vi "Robot Main.vi"() -> ()   [LabVIEW 2014]
doc: "This VI implements the framework and scheduler for your robotics program. It should not be necessary to modify the framework. You are expected to add your code to the VIs called from Robot Main - the ones located in the Team Code folder within the project."
uses:
  <vilib>/Rock Robotics/WPI/MotorControl/WPI_MotorControlDeviceRef.ctl
  <vilib>/Rock Robotics/WPI/MotorControl/WPI_MotorControlType.ctl
  <vilib>/Rock Robotics/SystemInterfaces/Typedef/FPGA_TypedefDigitalModule.ctl
  <vilib>/Rock Robotics/SystemInterfaces/DIO/FPGA_DIOPWMChannel.ctl
  <vilib>/Rock Robotics/WPI/PWM/WPI_PWMDeadband.ctl
  <vilib>/Rock Robotics/WPI/CAN/Jaguar/SubVIs/WPI_CANJaguar_ControlMode.ctl
  <vilib>/Rock Robotics/WPI/CAN/TalonSRX/WPI_CANTalonSRX_APIControlMode.ctl
  <vilib>/Rock Robotics/WPI/PWM/WPI_PWMTransform_ConPane.ctl
  <vilib>/Rock Robotics/WPI/Switch/WPI_SwitchDevRef.ctl
  <vilib>/Rock Robotics/SystemInterfaces/DIO/FPGA_DIOChannel.ctl
  <vilib>/Rock Robotics/SystemInterfaces/Counter/FPGA_CounterCtrSystemIndex.ctl
  <vilib>/Rock Robotics/SystemInterfaces/AI/FPGA_AIChannel.ctl
  <vilib>/Rock Robotics/WPI/Joystick/WPI_JoystickDeviceEnum.ctl
  <vilib>/Rock Robotics/WPI/MotorControl/WPI_MotorControlOpen Talon.vi
  <vilib>/Rock Robotics/WPI/Switch/WPI_SwitchOpenLimit.vi
  <vilib>/Rock Robotics/WPI/MotorControl/WPI_MotorControlOpen Victor.vi
  <vilib>/Rock Robotics/WPI/Counter/WPI_CounterDigitalInputToDigitalSource.vi
  <vilib>/Rock Robotics/WPI/RobotDrive/WPI_RobotDriveOpen4MotorWithVictor.vi
  Robot Global Data.vi
panel:
  in  "Gains DOWN":cluster{"P":dbl, "I":dbl, "D":dbl}={"P"=0.15555, "I"=5.6e-07, "D"=0.0}
  out "all currents (A)":dbl[](array[numeric])
  in  "Lift Deadband":dbl=0.1
  in  "Manual?":bool
  out "Distance":dbl
  out "Tolerable?":bool
  in  "Limit":dbl=0.666
  in  "Gains":cluster{"P":dbl, "I":dbl, "D":dbl}={"P"=0.15555, "I"=5.6e-07, "D"=0.0}
  in  "Limit Switches":T5={"Lift Top"={"DevStatus"={"status"=FALSE, "code"=0, "source"=""}, "DIO Channel"=enum."Invalid", "Controller"=enum."Controller 1", "CntIndex"=enum."Invalid", "Normally Closed"=FALSE}, "Lift Bottom"={"DevStatus"={"status"=FALSE, "code"=0, "source"=""}, "DIO Channel"=enum."Invalid", "Controller"=enum."Controller 1", "CntIndex"=enum."Invalid", "Normally Closed"=FALSE}, "Gripper 1"={"DevStatus"={"status"=FALSE, "code"=0, "source"=""}, "DIO Channel"=enum."Invalid", "Controller"=enum."Controller 1", "CntIndex"=enum."Invalid", "Normally Closed"=FALSE}, "Gripper 2"={"DevStatus"={"status"=FALSE, "code"=0, "source"=""}, "DIO Channel"=enum."Invalid", "Controller"=enum."Controller 1", "CntIndex"=enum."Invalid", "Normally Closed"=FALSE}}
  in  "Motors":T14
  # "P = 7\nI = 2.5E -5"
  # "devided gains by 45"
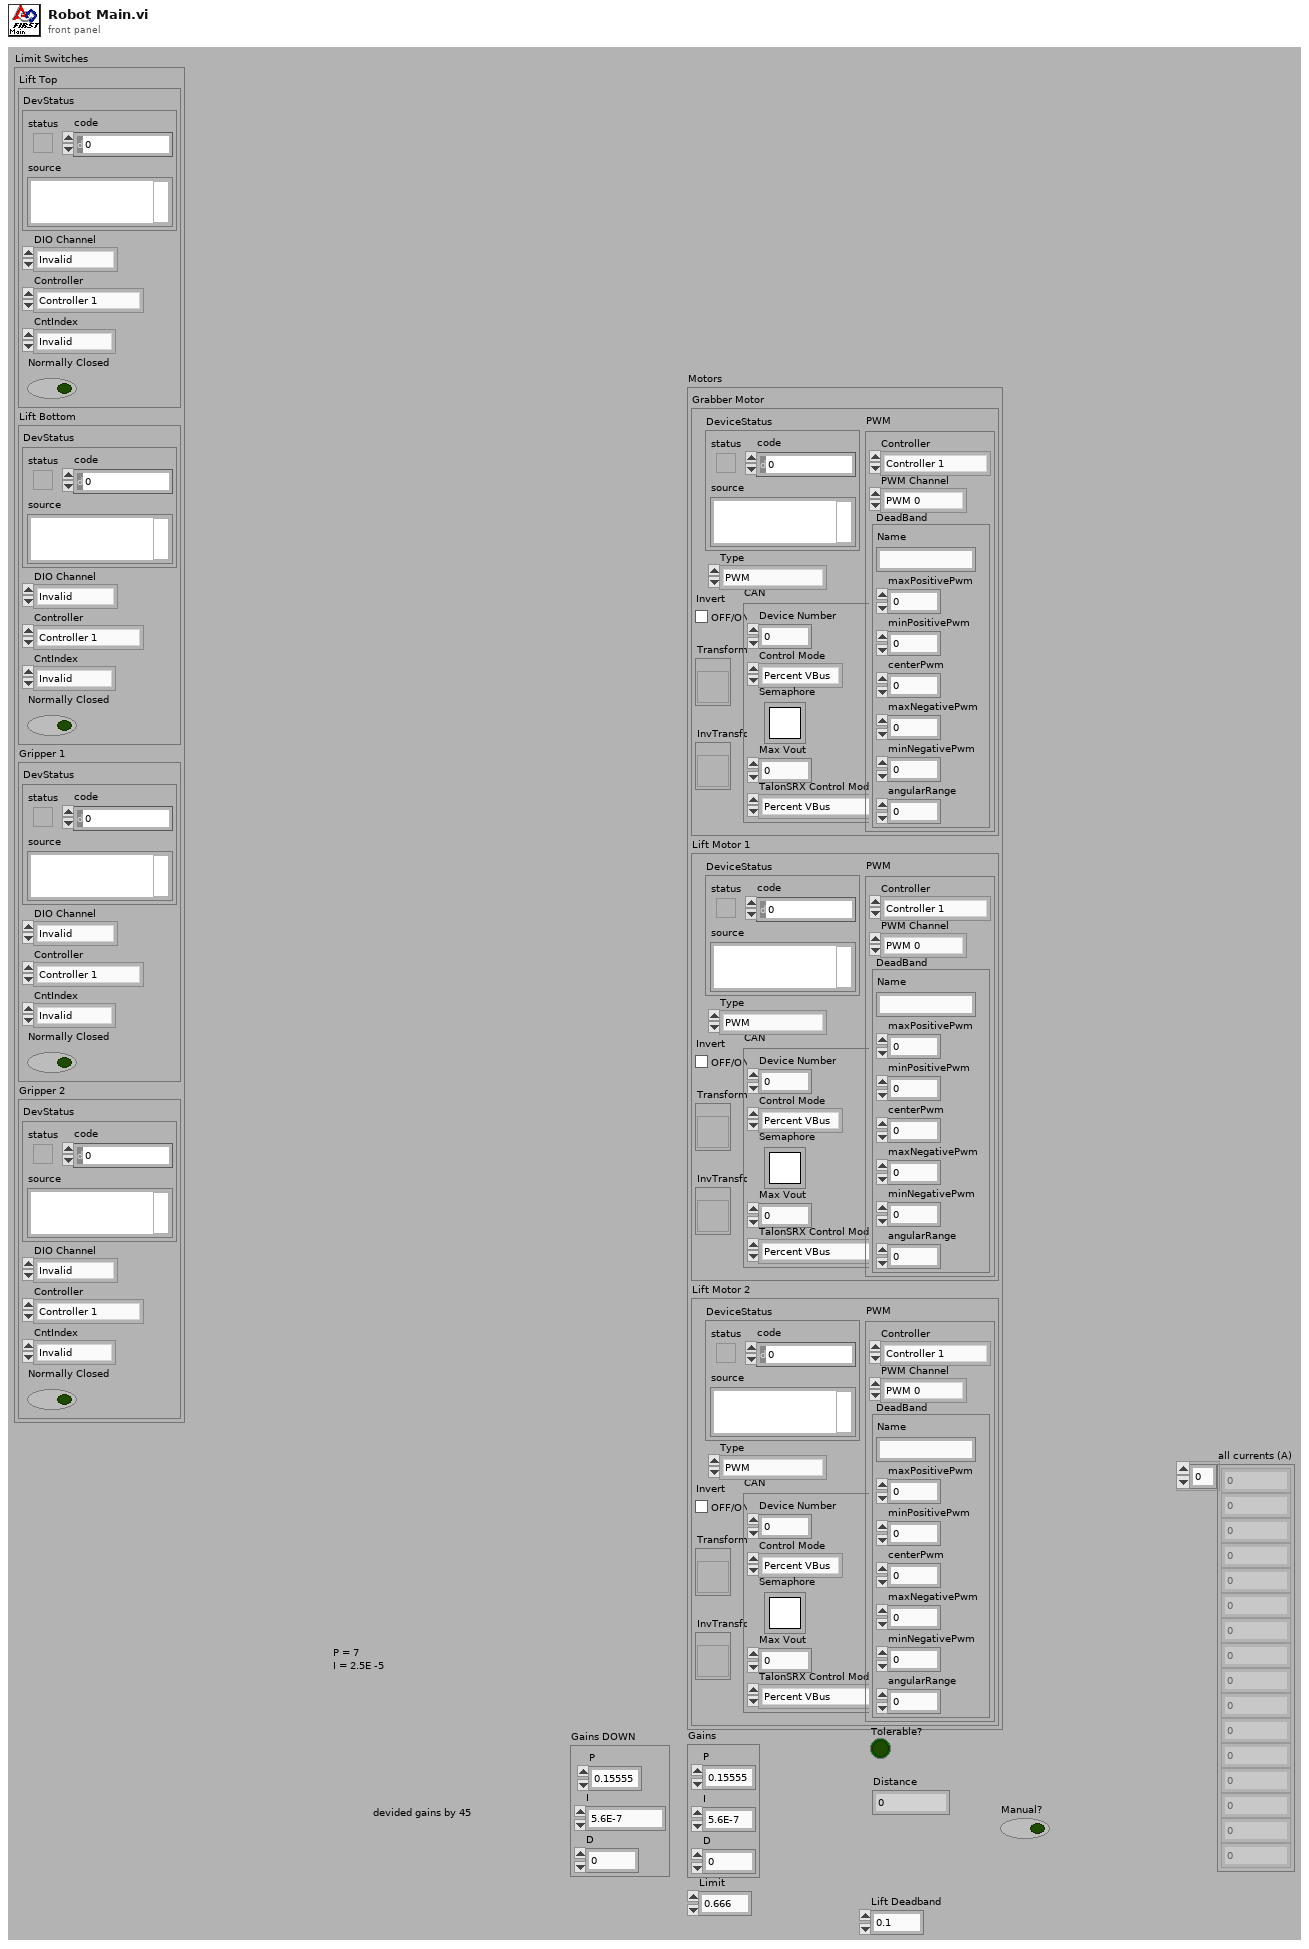
[diagram p1: front panel]
types:
  T1 = typedef "WPI_SwitchDevRef.ctl" = cluster{"DevStatus":errorcluster, "DIO Channel":T2, "Controller":T3, "CntIndex":T4, "Normally Closed":bool}
  T2 = typedef "FPGA_DIOChannel.ctl" = enum8{"DIO 0", "DIO 1", "DIO 2", "DIO 3", "DIO 4", "DIO 5", "DIO 6", "DIO 7", "DIO 8", "DIO 9", "DIO MXP 0", "DIO MXP 1", "DIO MXP 2", "DIO MXP 3", "DIO MXP 4", "DIO MXP 5", "DIO MXP 6", "DIO MXP 7", "DIO MXP 8", "DIO MXP 9", "DIO MXP 10", "DIO MXP 11", "DIO MXP 12", "DIO MXP 13", "DIO MXP 14", "DIO MXP 15", "Invalid"}
  T3 = typedef "FPGA_TypedefDigitalModule.ctl" = enum16{"Controller 1"}
  T4 = typedef "FPGA_CounterCtrSystemIndex.ctl" = enum8{"Ctr 0", "Ctr 1", "Ctr 2", "Ctr 3", "Ctr 4", "Ctr 5", "Ctr 6", "Ctr 7", "Invalid"}
  T5 = cluster{"Lift Top":T1, "Lift Bottom":T1, "Gripper 1":T1, "Gripper 2":T1}
  T6 = typedef "WPI_MotorControlDeviceRef.ctl" = cluster{"DeviceStatus":errorcluster, "Type":T7, "PWM":cluster{"Controller":T3, "PWM Channel":T8, "DeadBand":T9}, "CAN":cluster{"Device Number":u8, "Control Mode":T10, "Semaphore":T11, "Max Vout":dbl, "TalonSRX Control Mode":T12}, "Invert":bool, "TransformRef":T13, "InvTransformRef":T13}
  T7 = typedef "WPI_MotorControlType.ctl" = enum16{"PWM", "CAN", "CANTalonSRX"}
  T8 = typedef "FPGA_DIOPWMChannel.ctl" = enum8{"PWM 0", "PWM 1", "PWM 2", "PWM 3", "PWM 4", "PWM 5", "PWM 6", "PWM 7", "PWM 8", "PWM 9", "PWM MXP 0", "PWM MXP 1", "PWM MXP 2", "PWM MXP 3", "PWM MXP 4", "PWM MXP 5", "PWM MXP 6", "PWM MXP 7", "PWM MXP 8", "PWM MXP 9", "Invalid"}
  T9 = typedef "WPI_PWMDeadband.ctl" = cluster{"Name":string, "maxPositivePwm":i32, "minPositivePwm":i32, "centerPwm":i32, "maxNegativePwm":i32, "minNegativePwm":i32, "angularRange":u16}
  T10 = typedef "WPI_CANJaguar_ControlMode.ctl" = enum8{"Percent VBus", "Current", "Speed", "Position", "Voltage"}
  T11 = typedef "Semaphore RefNum" = refnum<k1>
  T12 = typedef "WPI_CANTalonSRX_APIControlMode.ctl" = enum8{"Percent VBus", "Speed", "Position", "Slave", "Unchanged / Invalid"}
  T13 = typedef "WPI_PWMTransform_ConPane.ctl" = refnum<vi>
  T14 = cluster{"Grabber Motor":T6, "Lift Motor 1":T6, "Lift Motor 2":T6}
  T15 = typedef "WPI_JoystickDeviceEnum.ctl" = enum16{"USB 0", "USB 1", "USB 2", "USB 3", "USB 4", "USB 5"}
  T16 = typedef "FPGA_AIChannel.ctl" = enum8{"AI 0", "AI 1", "AI 2", "AI 3", "AI MXP 0", "AI MXP 1", "AI MXP 2", "AI MXP 3", "Invalid"}
  T17 = typedef "WPI_DigitalInputDevRef.ctl" = cluster{"DevStatus":errorcluster, "DIO Channel":T2, "Controller":T3}
  T18 = typedef "WPI_JoystickDevRef.ctl" = cluster{"Device":T15}
  T19 = typedef "FPGA_CounterEncoderSourceConvertionLVSourceType.ctl" = cluster{"DevStatus":errorcluster, "AnalogTriggerMode?":bool, "DigitalMode":cluster{"Controller":T3, "DIO Channel":T20}, "AnalogTriggerMode":cluster{"AnalogTriggerIndex":T21, "OutputType":T22}}
  T20 = typedef "FPGA_DIODigitalSourceChannel.ctl" = enum8{"DIO 0", "DIO 1", "DIO 2", "DIO 3", "DIO 4", "DIO 5", "DIO 6", "DIO 7", "DIO 8", "DIO 9", "DIO MXP 0", "DIO MXP 1", "DIO MXP 2", "DIO MXP 3", "DIO MXP 4", "DIO MXP 5", "DIO MXP 6", "DIO MXP 7", "DIO MXP 8", "DIO MXP 9", "DIO MXP 10", "DIO MXP 11", "DIO MXP 12", "DIO MXP 13", "DIO MXP 14", "DIO MXP 15", "Disabled"}
  T21 = typedef "FPGA_AnalogTriggerIndex.ctl" = enum8{"Trig 0", "Trig 1", "Trig 2", "Trig 3", "Trig 4", "Trig 5", "Trig 6", "Trig 7", "Invalid"}
  T22 = typedef "FPGA_AnalogTriggerOutType.ctl" = enum16{"InWindow", "TriggerState", "Rising", "Falling"}
  T23 = typedef "WPI_PotentiometerDevRef.ctl" = cluster{"DevStatus":errorcluster, "Controller":T24, "Analog Channel":T16, "Invert Output":bool}
  T24 = typedef "FPGA_TypedefAnalogModule.ctl" = enum16{"Controller 1"}
  T25 = typedef "WPI_EncoderDevRef.ctl" = cluster{"DevStatus":errorcluster, "EncoderIndex":T26, "CounterIndex":T4, "DistancePerCount":dbl, "Decoding Type":T27}
  T26 = typedef "FPGA_EncoderIdx.ctl" = enum8{"Enc 0", "Enc 1", "Enc 2", "Enc 3", "Enc 4", "Enc 5", "Enc 6", "Enc 7", "Invalid"}
  T27 = typedef "WPI_EncoderType.ctl" = enum16{"1x", "2x", "4x"}
  T28 = typedef "WPI_RobotDriveDevRef.ctl" = cluster{"DevStatus":errorcluster, "Motors[]":T6[], "Square Inputs":bool, "Max Output":dbl}
  T29 = typedef "WPI_DriverStationRobotMode2.ctl" = enum16{"Autonomous Disabled", "Autonomous Enabled", "Teleop Disabled", "Teleop Enabled", "Disconnected", "Finish", "Test Disabled", "Test Enabled", "Emergency Stopped"}
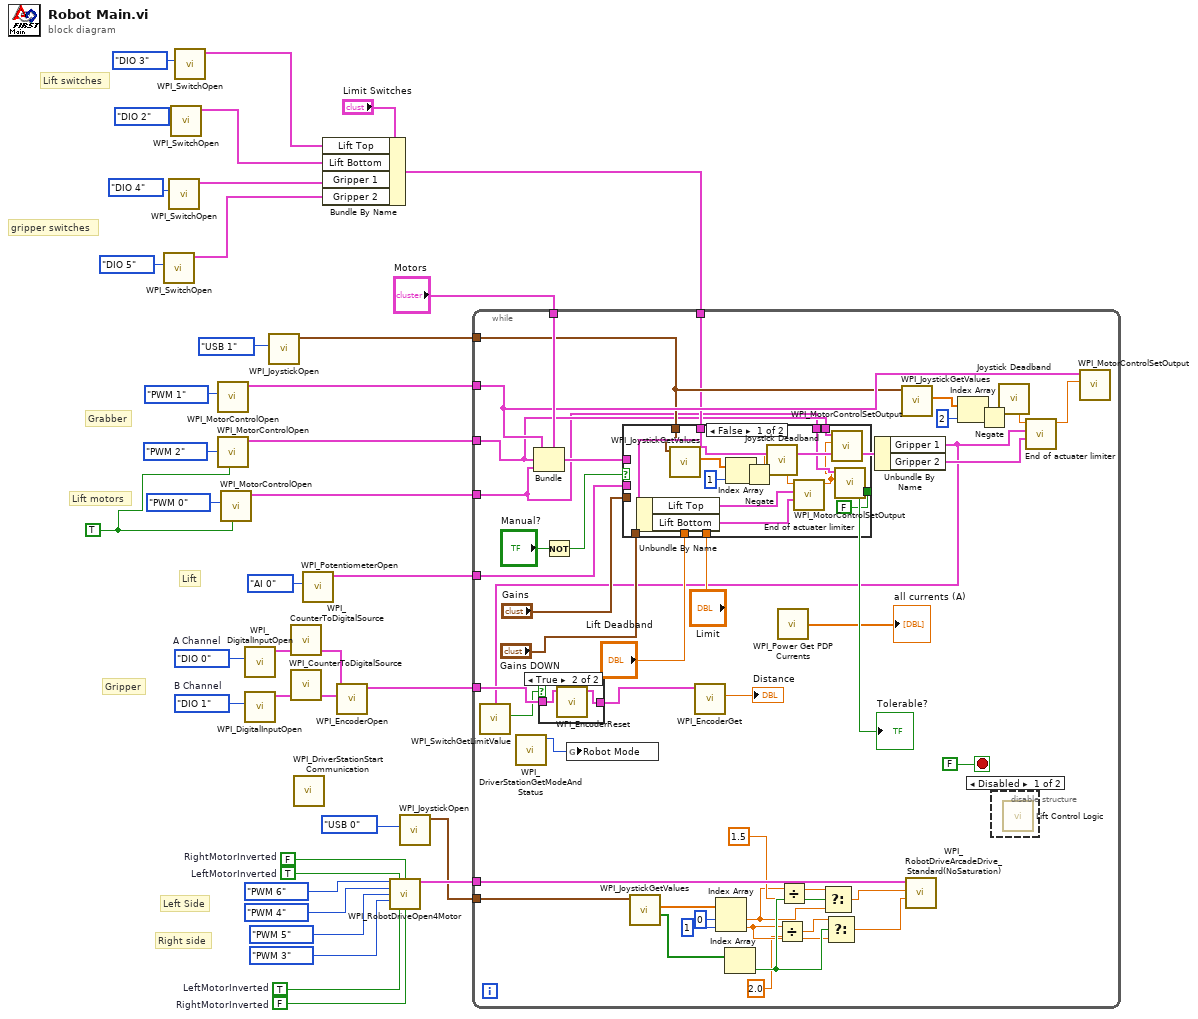
[diagram p0: block diagram]
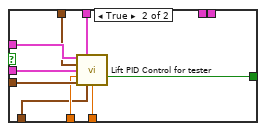
[diagram p4: hidden frame]
diagram:
  w5 = FALSE  # RightMotorInverted
  w4 = TRUE  # LeftMotorInverted
  w11 = TRUE  # LeftMotorInverted
  w10 = FALSE  # RightMotorInverted
  w17 = FPGA_DIOChannel."DIO 1"  # B Channel
  w16 = FPGA_DIOChannel."DIO 0"  # A Channel
  w18 = TRUE ("Invert")
  # "Right side"
  # "Left Side"
  # "Gripper"
  # "gripper switches"
  # "Lift switches"
  # "Grabber"
  # "Lift motors"
  # "Lift"
  n1 = call-poly <vilib>:"WPI_SwitchOpen.vi"("DIO Channel"=FPGA_DIOChannel."DIO 5") -> ("SwitchDevRef"=w21:T1)  [unwired: 9 in, 1 out]
  n2 = call-poly <vilib>:"WPI_SwitchOpen.vi"("DIO Channel"=FPGA_DIOChannel."DIO 4") -> ("SwitchDevRef"=w20:T1)  [unwired: 9 in, 1 out]
  n3 = call-poly <vilib>:"WPI_SwitchOpen.vi"("DIO Channel"=FPGA_DIOChannel."DIO 2") -> ("SwitchDevRef"=w22:T1)  [unwired: 9 in, 1 out]
  n4 = call-poly <vilib>:"WPI_SwitchOpen.vi"("DIO Channel"=FPGA_DIOChannel."DIO 3") -> ("SwitchDevRef"=w23:T1)  [unwired: 9 in, 1 out]
  n5 = call-poly <vilib>:"WPI_MotorControlOpen.vi"("PWM Channel"=FPGA_DIOPWMChannel."PWM 1") -> ("MotorControlDeviceRef"=w36:T6)  [unwired: 9 in, 1 out]
  n6 = call-poly <vilib>:"WPI_MotorControlOpen.vi"("Invert"=w18, "PWM Channel"=FPGA_DIOPWMChannel."PWM 2") -> ("MotorControlDeviceRef"=w35:T6)  [unwired: 8 in, 1 out]
  n7 = call-poly <vilib>:"WPI_MotorControlOpen.vi"("Invert"=w18, "PWM Channel"=FPGA_DIOPWMChannel."PWM 0") -> ("MotorControlDeviceRef"=w34:T6)  [unwired: 8 in, 1 out]
  n8 = call <vilib>:"WPI_DigitalInputOpen.vi"("DIO Channel"=w16) -> ("DigitalInputDevRef"=w13:T17)  [unwired: 2 in, 8 out]
  n9 = call <vilib>:"WPI_DigitalInputOpen.vi"("DIO Channel"=w17) -> ("DigitalInputDevRef"=w14:T17)  [unwired: 2 in, 8 out]
  n10 = call <vilib>:"WPI_JoystickOpen.vi"("JoystickDevice"=WPI_JoystickDeviceEnum."USB 1") -> ("JoystickDevRef"=w31:T18)  [unwired: 10 in]
  n11 = call-poly <vilib>:"WPI_CounterToDigitalSource.vi"("DigitalInputDevRef"=w13) -> ("Digital Source"=w12:T19)  [unwired: 6 out]
  n12 = call-poly <vilib>:"WPI_CounterToDigitalSource.vi"("DigitalInputDevRef"=w14) -> ("Digital Source"=w15:T19)  [unwired: 6 out]
  n13 = call <vilib>:"WPI_DriverStationStart Communication.vi"() -> ()  [unwired: 12 in]
  n14 = call <vilib>:"WPI_PotentiometerOpen.vi"("Analog Channel"=FPGA_AIChannel."AI 0") -> ("PotDevRef"=w33:T23)  [unwired: 9 in, 1 out]
  n15 = Bundle By Name(cluster="Limit Switches", "Lift Top"=w23, "Lift Bottom"=w22, "Gripper 1"=w20, "Gripper 2"=w21) -> (w19:T5)
  n16 = call <vilib>:"WPI_EncoderOpen.vi"("BSource"=w15, "ASource"=w12) -> ("EncoderDevRef"=w30:T25)  [unwired: 6 in, 3 out]
  n17 = call-poly <vilib>:"WPI_RobotDriveOpen4Motor.vi"("Rear Left Motor"=FPGA_DIOPWMChannel."PWM 6", "Rear Left Motor Inverted"=w11, "Rear Right Motor Inverted"=w10, "Rear Right Motor"=FPGA_DIOPWMChannel."PWM 4", "Front Left Motor"=FPGA_DIOPWMChannel."PWM 5", "Front Right Motor"=FPGA_DIOPWMChannel."PWM 3", "Front Left Motor Inverted"=w4, "Front Right Motor Inverted"=w5) -> ("RobotDriveDevRef"=w3:T28)  [unwired: 6 in, 1 out]
  n18 = call <vilib>:"WPI_JoystickOpen.vi"("JoystickDevice"=WPI_JoystickDeviceEnum."USB 0") -> ("JoystickDevRef"=w1:T18)  [unwired: 10 in]
  n19 = while {
    tunnel: w36 -> [w77]
    tunnel: w35 -> [w74]
    tunnel: w34 -> [w73]
    tunnel: w33 -> [w82]
    tunnel: w31 -> [w76]
    tunnel: w30 -> [w46]
    tunnel: "Motors" -> [w84]
    tunnel: w19 -> [w75]
    tunnel: w3 -> [w58]
    tunnel: w1 -> [w57]
    stop <- FALSE stop-if-true
    n20 = call <vilib>:"WPI_DriverStationGetModeAndStatus.vi"() -> ("Robot Mode"=w85:T29)  [unwired: 10 in, 1 out]
    n21 = Bundle(cluster=w84, "Grabber Motor"=w77, "Lift Motor 1"=w74, "Lift Motor 2"=w73) -> (w83:T14)
    n22 = Not(x="Manual?") -> (.not. x?=w71:bool)
    n23 = global write "Robot Global Data.vi" "Robot Mode"(w85) -> ()
    n24 = case shown="False" w71 {
      tunnel: w83 -> [_ w110]
      tunnel: w82 -> [_ w109]
      tunnel: "Gains" -> [_ w108]
      tunnel: "Limit" -> [_ w107]
      tunnel: [FALSE ("Tolerable?") w106] -> w79
      tunnel: w76 -> [w94 w105]
      tunnel: w75 -> [w95 w104]
      tunnel: w74 -> [w93 _]
      tunnel: w73 -> [w92 _]
      tunnel: "Lift Deadband" -> [_ w103]
      tunnel: "Gains DOWN" -> [_ w102]
      frame False {
        n25 = Unbundle By Name(w95) -> ("Lift Top"=w97:T1, "Lift Bottom"=w96:T1)
        n26 = call <vilib>:"WPI_JoystickGetValues.vi"("JoystickDevRef"=w94) -> ("Axes"=w101:dbl[])  [unwired: 6 in, 4 out]
        n27 = Index Array(array=w101, index=1) -> (element=w98:dbl)
        n28 = Negate(x=w98) -> (-x=w89:dbl)
        n29 = call "Joystick Deadband.vi"("Joystick Value"=w89) -> ("Joystick Output"=w99:dbl)  [unwired: 1 in]
        n30 = call "End of actuater limiter.vi"("Lower limit switch"=w96, "Upper limit switch"=w97, "Motor input"=w99) -> ("Motor output"=w91:dbl)  [unwired: 8 in]
        n31 = call <vilib>:"WPI_MotorControlSetOutput.vi"("Output"=w91, "MotorControlDevRef"=w93) -> ()  [unwired: 7 in, 3 out]
        n32 = call <vilib>:"WPI_MotorControlSetOutput.vi"("Output"=w91, "MotorControlDevRef"=w92) -> ()  [unwired: 7 in, 3 out]
      }
      frame True {
        n33 = call "Lift PID Control for tester.vi"("Motors DevRefs IN"=w110, "Limit Switches"=w104, "Operator Gamepad"=w105, "Lift Potentionmeter"=w109, "Lift Deadband"=w103, "Gains UP"=w108, "Gains DOWN"=w102, "Limit"=w107) -> ("Tolerable?"=w106:bool)  [unwired: 6 in, 1 out]
      }
    }
    "Tolerable?" <- w79
    n34 = call <vilib>:"WPI_JoystickGetValues.vi"("JoystickDevRef"=w57) -> ("Buttons"=w53:bool[], "Axes"=w61:dbl[])  [unwired: 6 in, 3 out]
    n35 = Index Array(array=w61, index #1=0 ("index"), index #2=1 ("index")) -> (element #1=w42:dbl, element #2=w50:dbl)
    n36 = Index Array(array=w53) -> (element=w52:bool)  [unwired: 1 in]
    n37 = Divide(x=w50, y=2.0) -> (x/y=w49:dbl)
    n38 = call <vilib>:"WPI_Power Get PDP Currents.vi"() -> ("all currents (A)"=→"all currents (A)":dbl[])  [unwired: 13 in, 2 out]
    n39 = Divide(x=w42, y=1.5) -> (x/y=w51:dbl)
    n40 = Select(t=w51, s=w52, f=w42) -> (s? t:f=w55:dbl)
    n41 = Select(t=w49, s=w52, f=w50) -> (s? t:f=w54:dbl)
    n42 = Unbundle By Name(w75) -> ("Gripper 1"=w44:T1, "Gripper 2"=w63:T1)
    n43 = call <vilib>:"WPI_SwitchGetLimitValue.vi"("SwitchDevRef"=w44) -> ("Switch Pressed"=w43:bool)  [unwired: 8 in, 2 out]
    n44 = case shown="True" w43 {
      tunnel: [w86 w88] -> w45
      tunnel: w46 -> [w86 w87]
      frame False {
      }
      frame True {
        n45 = call <vilib>:"WPI_EncoderReset.vi"("EncoderDevRef"=w87) -> ("EncoderDevRef"=w88:T25)  [unwired: 9 in, 1 out]
      }
    }
    n46 = call <vilib>:"WPI_EncoderGet.vi"("EncoderDevRef"=w45) -> ("Distance"=→"Distance":dbl)  [unwired: 5 in, 5 out]
    n47 = call <vilib>:"WPI_JoystickGetValues.vi"("JoystickDevRef"=w76) -> ("Axes"=w67:dbl[])  [unwired: 6 in, 4 out]
    n48 = call <vilib>:"WPI_RobotDriveArcadeDrive_Standard(NoSaturation).vi"("Y axis value"=w54, "X axis value"=w55, "RobotDriveDevRef"=w58) -> ()  [unwired: 1 in, 8 out]
    n49 = Index Array(array=w67, index=2) -> (element=w64:dbl)
    n50 = Negate(x=w64) -> (-x=w41:dbl)
    n51 = disable-structure shown="Disabled" {
      frame Disabled {
        n52 = call "Lift Control Logic.vi"() -> ()  [unwired: 12 in, 4 out]
      }
      frame Enabled {
      }
    }
    n53 = call "Joystick Deadband.vi"("Joystick Value"=w41) -> ("Joystick Output"=w65:dbl)  [unwired: 1 in]
    n54 = call "End of actuater limiter.vi"("Lower limit switch"=w63, "Upper limit switch"=w44, "Motor input"=w65) -> ("Motor output"=w56:dbl)  [unwired: 8 in]
    n55 = call <vilib>:"WPI_MotorControlSetOutput.vi"("Output"=w56, "MotorControlDevRef"=w77) -> ()  [unwired: 7 in, 3 out]
  }
